vi "Standalone REST.vi"() -> ()   [LabVIEW 2023]
uses:
  Log/Log_Level.ctl
  API Message/API Message.lvclass
  Log/Log_Facilities.ctl
  Response/Standard Response Messages.ctl
  5ff5fe4d-644e-42b3-82e9-72adbb7d47a0.vi
  701e6035-b014-4147-aab3-b3ce1f9fae1e.vi
  5a67b58a-d501-4dc3-8558-0c804d545b7c.vi
  e8db4eca-cc96-4f6d-a0d1-e29095bc51eb.vi
  1441fe33-22a0-4e61-8bdf-aaa6b22bb0fa.vi
  c70d4357-6874-4551-bf72-0a3070db1cee.vi
  baea4f90-ed66-40c9-855f-b5689293d002.vi
  5ff5fe4d-644e-42b3-82e9-72adbb7d47a0.vi/bf0030c7-b76b-4182-9f9e-16cd2e366061.vi
  701e6035-b014-4147-aab3-b3ce1f9fae1e.vi/bf0030c7-b76b-4182-9f9e-16cd2e366061.vi
  5a67b58a-d501-4dc3-8558-0c804d545b7c.vi/bf0030c7-b76b-4182-9f9e-16cd2e366061.vi
  e8db4eca-cc96-4f6d-a0d1-e29095bc51eb.vi/bf0030c7-b76b-4182-9f9e-16cd2e366061.vi
  1441fe33-22a0-4e61-8bdf-aaa6b22bb0fa.vi/bf0030c7-b76b-4182-9f9e-16cd2e366061.vi
  c70d4357-6874-4551-bf72-0a3070db1cee.vi/bf0030c7-b76b-4182-9f9e-16cd2e366061.vi
  baea4f90-ed66-40c9-855f-b5689293d002.vi/bf0030c7-b76b-4182-9f9e-16cd2e366061.vi
  Request/Get Request.vi
  Response/Set Body.vi
  Response/Set Content Type.vi
  Response/Set Status Code.vi
  Response/Send.vi
  <vilib>/Platform/browser.llb/Open URL in Default Browser (string).vi
  Request/Request.lvclass
  Response/Response.lvclass
  Log/Log.lvclass
  Server/Server.lvclass
panel:
  in  "Test 2":bool
  in  "Read 1":bool
  in  "Thing 2":string="Value 2"
  in  "Thing 1":string="Value 1"
  in  "stop":bool
  # "These buttons simply open the system default browser to \nGET the value from the REST endpoints for these 2 strings"
  # "These endpoints would normally consumed by another\nprogram, not a browser."
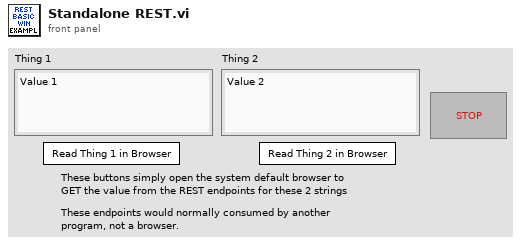
[diagram p1: front panel]
types:
  T1 = typedef "Log.lvclass/Log_Level.ctl" = enum16{"none", "info", "trace", "warn", "error", "fatal"}
  T2 = enum32{"invalid app kind", "Development System", "Run Time System", "Student Edition", "Embedded LabVIEW", "Evaluation", "Custom"}
  T3 = typedef "Log.lvclass/Log_Facilities.ctl" = string
  T4 = typedef "Request.ctl" = cluster{"Method":string, "URI":string, "Protocol":string, "Raw Path":string, "Query":string, "Fragment":string, "Raw Body":string, "Headers":variant, "Parameters":variant, "Body":variant, "Raw Header":string, "Path":string[]}
  T5 = typedef "Response.lvclass/Standard Response Messages.ctl" = u16
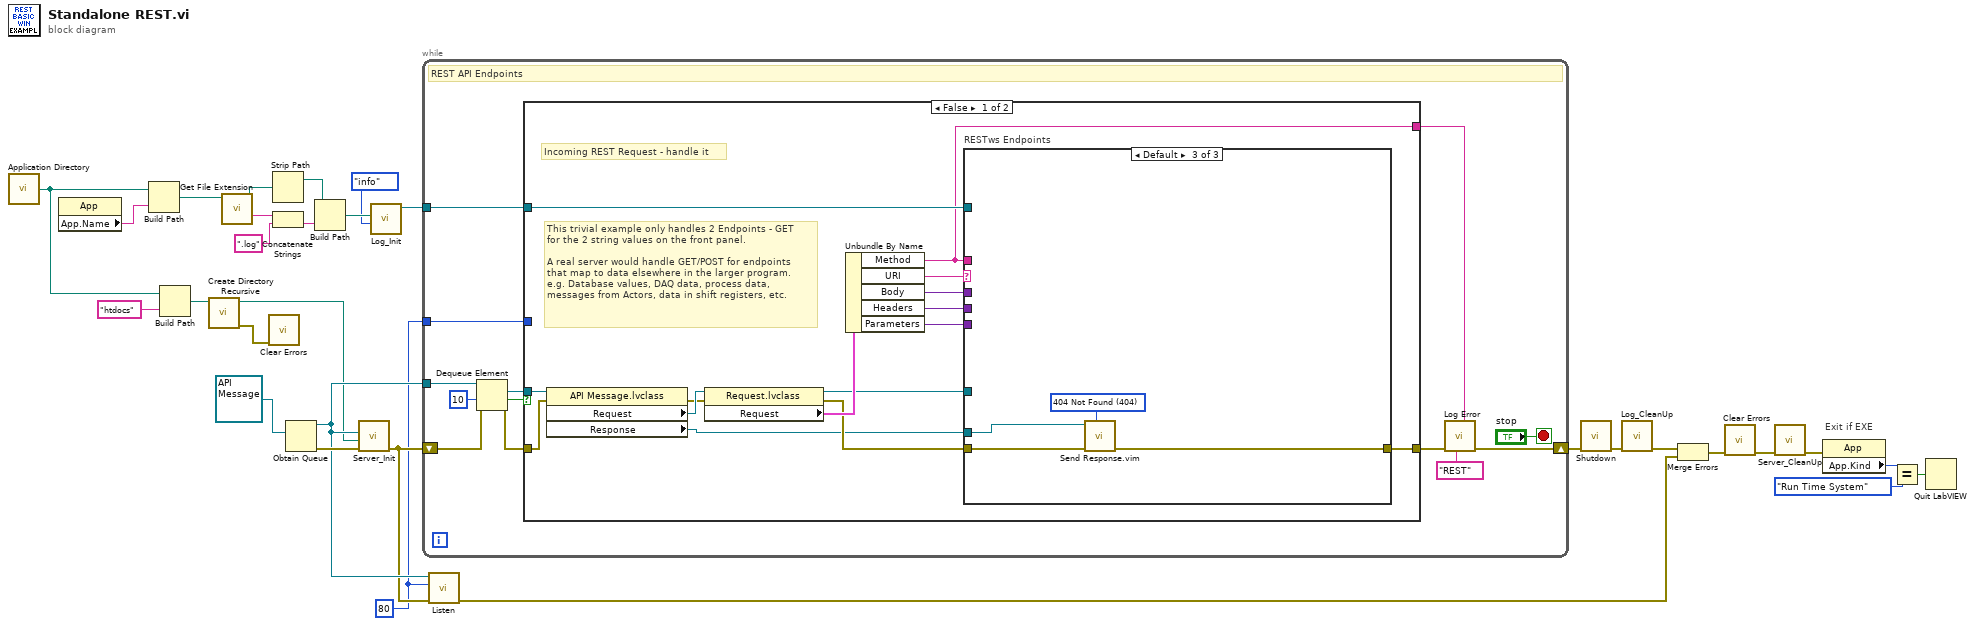
[diagram p0: block diagram]
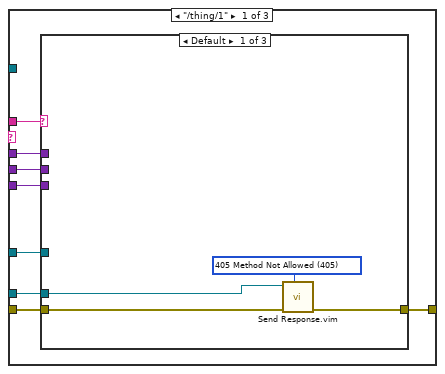
[diagram p2: hidden frame]
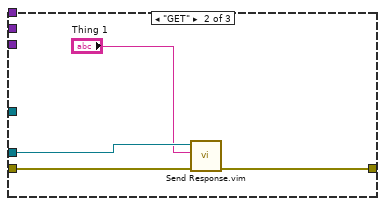
[diagram p3: hidden frame]
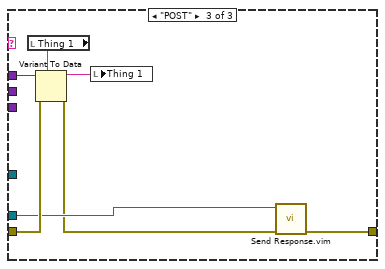
[diagram p4: hidden frame]
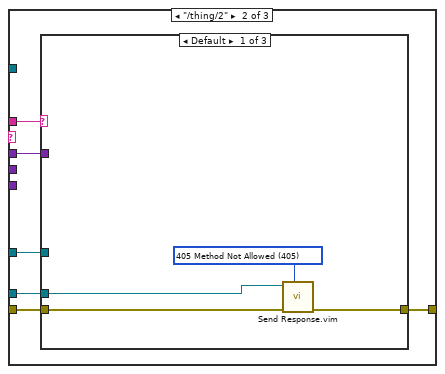
[diagram p5: hidden frame]
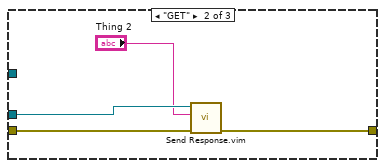
[diagram p6: hidden frame]
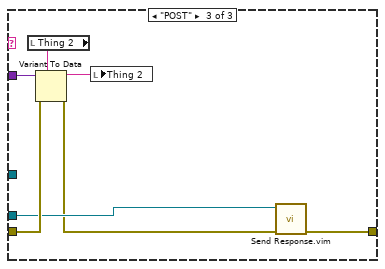
[diagram p7: hidden frame]
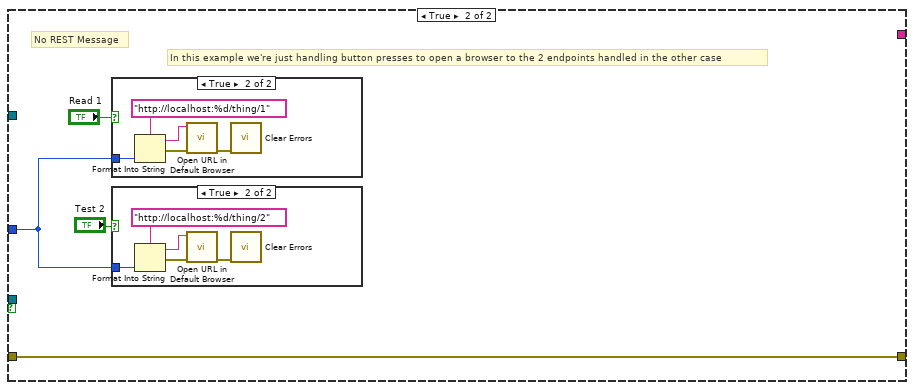
[diagram p8: hidden frame]
diagram:
  w4 = u16 80 ("Listen Port (80)")
  # "Exit if EXE"
  n1 = call <vilib>:"Application Directory.vi"() -> ("Application Directory"=w18:path)
  n2 = property class="App"() -> ("App.Name"=w13:string)  [unwired: 2 in, 2 out]
  n3 = Build Path(base path=w18, name or relative path=w13) -> (appended path=w15:path)
  n4 = Build Path(base path=w18, name or relative path="htdocs" ("section")) -> (appended path=w3:path)
  n5 = call <vilib>:"Create Directory Recursive.vi"("directory"=w3) -> ("error out"=w1:errorcluster, "directory copy"=w2:path)  [unwired: 4 in, 1 out]
  n6 = call <vilib>:"Get File Extension.vi"("file"=w15) -> ("filename without extension"=w23:string, "dup file"=w22:path)  [unwired: 6 in, 3 out]
  n7 = call <vilib>:"Clear Errors.vi"("error in (no error)"=w1) -> ()  [unwired: 5 in, 2 out]
  n8 = Strip Path(path=w22) -> (stripped path=w21:path)  [unwired: 1 out]
  n9 = Concatenate Strings(w23, ".log" ("section")) -> (w26:string)
  n10 = Obtain Queue(element data type=refnum<class "API Message.lvclass"> refnum ("API Message.lvclass")) -> (queue out=w16:refnum<queue>, error out=w20:errorcluster)  [unwired: 4 in, 1 out]
  n11 = Build Path(base path=w21, name or relative path=w26) -> (appended path=w25:path)
  n12 = call "Server_Init.vi"("error in (no error)"=w20, "Static Data Folder"=w2, "API Queue"=w16) -> ("error out"=w14:errorcluster)  [unwired: 7 in, 1 out]
  n13 = call "Log_Init.vi"("Level"=Log_Level."info", "Log File"=w25) -> ("reference out"=w10:refnum<class "Log.lvclass">)  [unwired: 8 in, 1 out]
  n14 = while "Send to RT" {
    shift-right: [w34] -> w8
    shift-left: w14 -> [w38]
    tunnel: w16 -> [w43]
    tunnel: w10 -> [w36]
    tunnel: w4 -> [w31]
    stop <- "stop" stop-if-true
    # "REST API Endpoints"
    n15 = Dequeue Element(queue=w43, timeout in ms (-1)=10, error in (no error)=w38) -> (element=w40:refnum<class "API Message.lvclass">, timed out?=w42:bool, error out=w41:errorcluster)  [unwired: 1 out]
    n16 = case shown="False" w42 {
      tunnel: w41 -> [w57 w110]
      tunnel: [w51 w110] -> w35
      tunnel: w40 -> [w58 _]
      tunnel: w36 -> [w47 _]
      tunnel: [w46 _] -> w32
      tunnel: w31 -> [_ w107]
      frame False {
        # "This trivial example only handles 2 Endpoints - GET\nfor the 2 string values on the front panel.\n\nA real server would handle GET/POST for endpoints\nthat map to data elsewhere in the larger program.\ne.g. Database values, DAQ data, process data, \nmessages from Actors, data in shift registers, etc."
        # "Incoming REST Request - handle it"
        n17 = property class="API Message.lvclass"(reference=w58, error in=w57) -> (error out=w55:errorcluster, "Request"=w56:refnum<class "Request.lvclass">, "Response"=w49:refnum<class "Response.lvclass">)  [unwired: 1 out]
        n18 = property class="Request.lvclass"(reference=w56, error in=w55) -> (reference out=w50:refnum<class "Request.lvclass">, error out=w52:errorcluster, "Request"=w54:T4)
        n19 = Unbundle By Name(w54) -> ("Method"=w46:string, "URI"=w53:string, "Body"=w48:variant, "Headers"=w45:variant, "Parameters"=w44:variant)
        n20 = case "RESTws Endpoints" shown="Default" w53 {
          tunnel: w52 -> [w65 w86 w105]
          tunnel: [w66 w87 w106] -> w51
          tunnel: w46 -> [w62 w83 _]
          tunnel: w50 -> [w64 w85 _]
          tunnel: w49 -> [w63 w84 w104]
          tunnel: w48 -> [w61 w82 _]
          tunnel: w47 -> [_ _ _]
          tunnel: w45 -> [w60 _ _]
          tunnel: w44 -> [w59 _ _]
          frame "/thing/1" {
            n21 = case shown="Default" w62 {
              tunnel: [w68 w73 w75] -> w66
              tunnel: w65 -> [w70 w74 w80]
              tunnel: w64 -> [_ _ _]
              tunnel: w63 -> [w69 w72 w78]
              tunnel: w61 -> [_ _ w81]
              tunnel: w60 -> [_ _ _]
              tunnel: w59 -> [_ _ _]
              frame Default {
                w67 = T5 405 items=["200 OK"=200, "201 Created"=201, "202 Accepted"=202, "203 Non-Authoritative Information"=203, "204 No Content"=204, "205 Reset Content"=205, "206 Partial Content"=206, "207 Multi-Status (WebDAV)"=207, "208 Already Reported (WebDAV)"=208, "226 IM Used (HTTP Delta encoding)"=226, "300 Multiple Choices"=300, "301 Moved Permanently"=301, "302 Found"=302, "303 See Other"=303, "304 Not Modified"=304, "305 Use Proxy Deprecated"=305, "307 Temporary Redirect"=307, "308 Permanent Redirect"=308, "400 Bad Request"=400, "401 Unauthorized"=401, "402 Payment Required"=402, "403 Forbidden"=403, "404 Not Found"=404, "405 Method Not Allowed"=405, "406 Not Acceptable"=406, "407 Proxy Authentication Required"=407, "408 Request Timeout"=408, "409 Conflict"=409, "410 Gone"=410, "411 Length Required"=411, "412 Precondition Failed"=412, "413 Content Too Large"=413, "414 URI Too Long"=414, "415 Unsupported Media Type"=415, "416 Range Not Satisfiable"=416, "417 Expectation Failed"=417, "418 I'm a teapot"=418, "421 Misdirected Request"=421, "422 Unprocessable Content (WebDAV)"=422, "423 Locked (WebDAV)"=423, "424 Failed Dependency (WebDAV)"=424, "425 Too Early Experimental"=425, "426 Upgrade Required"=426, "428 Precondition Required"=428, "429 Too Many Requests"=429, "431 Request Header Fields Too Large"=431, "451 Unavailable For Legal Reasons"=451, "500 Internal Server Error"=500, "501 Not Implemented"=501, "502 Bad Gateway"=502, "503 Service Unavailable"=503, "504 Gateway Timeout"=504, "505 HTTP Version Not Supported"=505, "506 Variant Also Negotiates"=506, "507 Insufficient Storage (WebDAV)"=507, "508 Loop Detected (WebDAV)"=508, "510 Not Extended"=510, "511 Network Authentication Required"=511] ("Status Codes")
                n22 = call "Send Response.vim"("Status Code (200=OK)"=w67, "Error In"=w70, "Response"=w69) -> ("Error Out"=w68:errorcluster)  [unwired: 8 in]
              }
              frame "GET" {
                n23 = call "Send Response.vim"("Error In"=w74, "Body (\"\")"="Thing 1", "Response"=w72) -> ("Error Out"=w73:errorcluster)  [unwired: 8 in]
              }
              frame "POST" {
                n24 = local read "Thing 1"() -> (w76:string)
                n25 = Variant To Data(error in=w80, type=w76, Variant=w81) -> (data=w79:string, error out=w77:errorcluster)
                n26 = local write "Thing 1"(w79) -> ()
                n27 = call "Send Response.vim"("Error In"=w77, "Response"=w78) -> ("Error Out"=w75:errorcluster)  [unwired: 9 in]
              }
            }
          }
          frame "/thing/2" {
            n28 = case shown="Default" w83 {
              tunnel: [w89 w94 w96] -> w87
              tunnel: w86 -> [w91 w95 w101]
              tunnel: w85 -> [_ _ _]
              tunnel: w84 -> [w90 w93 w99]
              tunnel: w82 -> [_ _ w102]
              frame Default {
                w88 = T5 405 items=["200 OK"=200, "201 Created"=201, "202 Accepted"=202, "203 Non-Authoritative Information"=203, "204 No Content"=204, "205 Reset Content"=205, "206 Partial Content"=206, "207 Multi-Status (WebDAV)"=207, "208 Already Reported (WebDAV)"=208, "226 IM Used (HTTP Delta encoding)"=226, "300 Multiple Choices"=300, "301 Moved Permanently"=301, "302 Found"=302, "303 See Other"=303, "304 Not Modified"=304, "305 Use Proxy Deprecated"=305, "307 Temporary Redirect"=307, "308 Permanent Redirect"=308, "400 Bad Request"=400, "401 Unauthorized"=401, "402 Payment Required"=402, "403 Forbidden"=403, "404 Not Found"=404, "405 Method Not Allowed"=405, "406 Not Acceptable"=406, "407 Proxy Authentication Required"=407, "408 Request Timeout"=408, "409 Conflict"=409, "410 Gone"=410, "411 Length Required"=411, "412 Precondition Failed"=412, "413 Content Too Large"=413, "414 URI Too Long"=414, "415 Unsupported Media Type"=415, "416 Range Not Satisfiable"=416, "417 Expectation Failed"=417, "418 I'm a teapot"=418, "421 Misdirected Request"=421, "422 Unprocessable Content (WebDAV)"=422, "423 Locked (WebDAV)"=423, "424 Failed Dependency (WebDAV)"=424, "425 Too Early Experimental"=425, "426 Upgrade Required"=426, "428 Precondition Required"=428, "429 Too Many Requests"=429, "431 Request Header Fields Too Large"=431, "451 Unavailable For Legal Reasons"=451, "500 Internal Server Error"=500, "501 Not Implemented"=501, "502 Bad Gateway"=502, "503 Service Unavailable"=503, "504 Gateway Timeout"=504, "505 HTTP Version Not Supported"=505, "506 Variant Also Negotiates"=506, "507 Insufficient Storage (WebDAV)"=507, "508 Loop Detected (WebDAV)"=508, "510 Not Extended"=510, "511 Network Authentication Required"=511] ("Status Codes")
                n29 = call "Send Response.vim"("Status Code (200=OK)"=w88, "Error In"=w91, "Response"=w90) -> ("Error Out"=w89:errorcluster)  [unwired: 8 in]
              }
              frame "GET" {
                n30 = call "Send Response.vim"("Error In"=w95, "Body (\"\")"="Thing 2", "Response"=w93) -> ("Error Out"=w94:errorcluster)  [unwired: 8 in]
              }
              frame "POST" {
                n31 = local read "Thing 2"() -> (w97:string)
                n32 = Variant To Data(error in=w101, type=w97, Variant=w102) -> (data=w100:string, error out=w98:errorcluster)
                n33 = local write "Thing 2"(w100) -> ()
                n34 = call "Send Response.vim"("Error In"=w98, "Response"=w99) -> ("Error Out"=w96:errorcluster)  [unwired: 9 in]
              }
            }
          }
          frame Default {
            w103 = T5 404 items=["200 OK"=200, "201 Created"=201, "202 Accepted"=202, "203 Non-Authoritative Information"=203, "204 No Content"=204, "205 Reset Content"=205, "206 Partial Content"=206, "207 Multi-Status (WebDAV)"=207, "208 Already Reported (WebDAV)"=208, "226 IM Used (HTTP Delta encoding)"=226, "300 Multiple Choices"=300, "301 Moved Permanently"=301, "302 Found"=302, "303 See Other"=303, "304 Not Modified"=304, "305 Use Proxy Deprecated"=305, "307 Temporary Redirect"=307, "308 Permanent Redirect"=308, "400 Bad Request"=400, "401 Unauthorized"=401, "402 Payment Required"=402, "403 Forbidden"=403, "404 Not Found"=404, "405 Method Not Allowed"=405, "406 Not Acceptable"=406, "407 Proxy Authentication Required"=407, "408 Request Timeout"=408, "409 Conflict"=409, "410 Gone"=410, "411 Length Required"=411, "412 Precondition Failed"=412, "413 Content Too Large"=413, "414 URI Too Long"=414, "415 Unsupported Media Type"=415, "416 Range Not Satisfiable"=416, "417 Expectation Failed"=417, "418 I'm a teapot"=418, "421 Misdirected Request"=421, "422 Unprocessable Content (WebDAV)"=422, "423 Locked (WebDAV)"=423, "424 Failed Dependency (WebDAV)"=424, "425 Too Early Experimental"=425, "426 Upgrade Required"=426, "428 Precondition Required"=428, "429 Too Many Requests"=429, "431 Request Header Fields Too Large"=431, "451 Unavailable For Legal Reasons"=451, "500 Internal Server Error"=500, "501 Not Implemented"=501, "502 Bad Gateway"=502, "503 Service Unavailable"=503, "504 Gateway Timeout"=504, "505 HTTP Version Not Supported"=505, "506 Variant Also Negotiates"=506, "507 Insufficient Storage (WebDAV)"=507, "508 Loop Detected (WebDAV)"=508, "510 Not Extended"=510, "511 Network Authentication Required"=511] ("Status Codes")
            n35 = call "Send Response.vim"("Status Code (200=OK)"=w103, "Error In"=w105, "Response"=w104) -> ("Error Out"=w106:errorcluster)  [unwired: 8 in]
          }
        }
      }
      frame True {
        # "In this example we're just handling button presses to open a browser to the 2 endpoints handled in the other case"
        # "No REST Message"
        n36 = case shown="True" "Read 1" {
          tunnel: w107 -> [_ w120]
          frame False {
          }
          frame True {
            n37 = Format Into String(format string="http://localhost:%d/thing/1", w120) -> (resulting string=w116:string, error out=w118:errorcluster)  [unwired: 2 in]
            n38 = call-poly <vilib>:"Open URL in Default Browser.vi"("error in (no error)"=w118, "URL"=w116) -> ("error out"=w117:errorcluster)  [unwired: 4 in, 1 out]
            n39 = call <vilib>:"Clear Errors.vi"("error in (no error)"=w117) -> ()  [unwired: 5 in, 2 out]
          }
        }
        n40 = case shown="True" "Test 2" {
          tunnel: w107 -> [_ w115]
          frame False {
          }
          frame True {
            n41 = Format Into String(format string="http://localhost:%d/thing/2", w115) -> (resulting string=w111:string, error out=w113:errorcluster)  [unwired: 2 in]
            n42 = call-poly <vilib>:"Open URL in Default Browser.vi"("error in (no error)"=w113, "URL"=w111) -> ("error out"=w112:errorcluster)  [unwired: 4 in, 1 out]
            n43 = call <vilib>:"Clear Errors.vi"("error in (no error)"=w112) -> ()  [unwired: 5 in, 2 out]
          }
        }
      }
    }
    n44 = call "Log Error.vi"("Context"=w32, "Facility (default)"=T3 "REST", "error in (no error)"=w35) -> ("error out"=w34:errorcluster)  [unwired: 8 in]
  }
  n45 = call "Listen.vi"("error in (no error)"=w14, "Listen Port (80)"=w4, "API Queue"=w16) -> ("error out"=w11:errorcluster)  [unwired: 8 in]
  n46 = call "Shutdown.vi"("error in (no error)"=w8) -> ("error out"=w7:errorcluster)  [unwired: 10 in]
  n47 = call "Log_CleanUp.vi"("error in (no error)"=w7) -> ("error out"=w9:errorcluster)  [unwired: 10 in]
  n48 = Merge Errors(w9, w11) -> (w12:errorcluster)
  n49 = call <vilib>:"Clear Errors.vi"("error in (no error)"=w12) -> ("error out"=w6:errorcluster)  [unwired: 5 in, 1 out]
  n50 = call "Server_CleanUp.vi"("error in (no error)"=w6) -> ("error out"=w5:errorcluster)  [unwired: 10 in]
  n51 = property class="App"(error in=w5) -> ("App.Kind"=w30:T2)  [unwired: 1 in, 2 out]
  n52 = Equal?(x=w30, y=T2."Run Time System" ("Application:Kind")) -> (x = y?=w28:bool)
  n53 = Quit LabVIEW(quit? (T)=w28) -> ()
